vi "cmd-ack-rebundler.vi"(11 "cmd-ack-in":T2) -> (3 "adam-chassis-cmd-ack":T3)   [LabVIEW 2024]
uses:
  controls/adam-5000-module-cmd-ack.ctl
  controls/adam-5000-chassis-cmd-ack.ctl
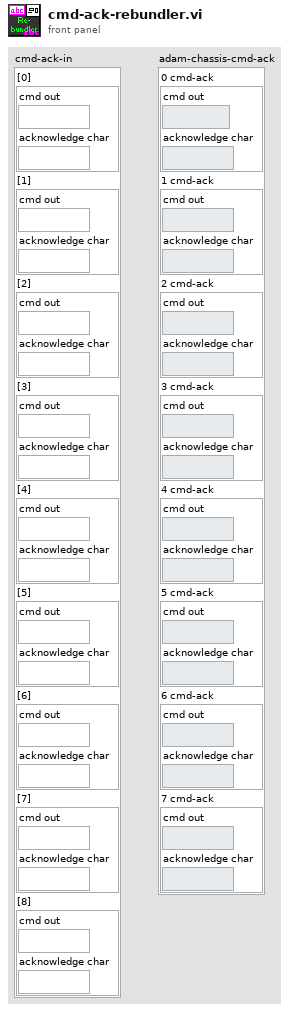
[diagram p1: front panel]
types:
  T1 = typedef "adam-5000-module-cmd-ack.ctl" = cluster{"cmd out":string, "acknowledge char":string}
  T2 = cluster{"[0]":T1, "[1]":T1, "[2]":T1, "[3]":T1, "[4]":T1, "[5]":T1, "[6]":T1, "[7]":T1, "[8]":T1}
  T3 = typedef "adam-5000-chassis-cmd-ack.ctl" = cluster{"0 cmd-ack":T1, "1 cmd-ack":T1, "2 cmd-ack":T1, "3 cmd-ack":T1, "4 cmd-ack":T1, "5 cmd-ack":T1, "6 cmd-ack":T1, "7 cmd-ack":T1}
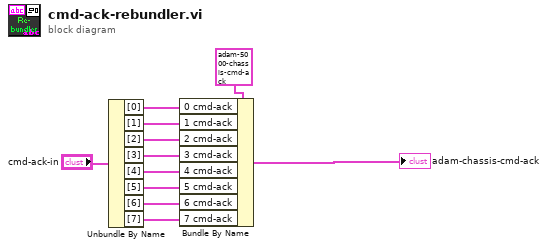
[diagram p0: block diagram]
diagram:
  n1 = Unbundle By Name("cmd-ack-in") -> ("[0]"=w2:T1, "[1]"=w3:T1, "[2]"=w6:T1, "[3]"=w7:T1, "[4]"=w8:T1, "[5]"=w9:T1, "[6]"=w10:T1, "[7]"=w11:T1)
  n2 = Bundle By Name(cluster=T3 {"0 cmd-ack"={"cmd out"="", "acknowledge char"=""}, "1 cmd-ack"={"cmd out"="", "acknowledge char"=""}, "2 cmd-ack"={"cmd out"="", "acknowledge char"=""}, "3 cmd-ack"={"cmd out"="", "acknowledge char"=""}, "4 cmd-ack"={"cmd out"="", "acknowledge char"=""}, "5 cmd-ack"={"cmd out"="", "acknowledge char"=""}, "6 cmd-ack"={"cmd out"="", "acknowledge char"=""}, "7 cmd-ack"={"cmd out"="", "acknowledge char"=""}} ("adam-chassis-cmd-ack"), "0 cmd-ack"=w2, "1 cmd-ack"=w3, "2 cmd-ack"=w6, "3 cmd-ack"=w7, "4 cmd-ack"=w8, "5 cmd-ack"=w9, "6 cmd-ack"=w10, "7 cmd-ack"=w11) -> (→"adam-chassis-cmd-ack":T3)
